vi "ReadParticleSizeSpectrum.vi"(1 "file path":path, 2 "Factor Size paramter":dbl=1.0) -> (0 "Particle Distribution Data":T1)   [LabVIEW 2013]
uses:
  ParticleDistributionData.ctl
  <vilib>/Platform/storage/lvStorage.llb/_openStorageWithRootAutoDetect.vi
  <vilib>/Platform/storage/lvStorage.llb/xStorage/xStorageSupp/ErrorOut.vi
  <vilib>/Platform/storage/lvStorage.llb/_queryPropPoly.vi
  <vilib>/Platform/storage/lvStorage.llb/_queryPropString.vi
  <vilib>/Platform/storage/lvStorage.llb/_queryGenericObjects.vi
  <vilib>/Platform/storage/lvStorage.llb/_loadAllDouble.vi
  <vilib>/Platform/storage/Storage.llb/Get Object Info.vi
  <vilib>/Platform/storage/Storage.llb/__closeStorageFromObject.vi
  <vilib>/imath/engines/lvmath2/RunTimeEngine/ErrorHandling/NIMS_Finalize Error.vi
  <vilib>/imath/engines/lvmath2/RunTimeEngine/IndexRead/NIMS M(S,$).vi
  <instcachedir>/0/NIMS M(S,$)_F24F360562DE41D8BE234322A2E15C65.lvgen/NIMS M(S,$)_F24F360562DE41D8BE234322A2E15C65_000.vi
  <vilib>/imathl/engines/lvmath/Functions/Error Handling/Create Error.vi
  <vilib>/imath/engines/lvmath2/RunTimeEngine/IndexRead/NIMS M(R2,$).vi
  <instcachedir>/0/NIMS M(R2,$)_AD8DC2FC79024024B2717E13B4A0EB4B.lvgen/NIMS M(R2,$)_AD8DC2FC79024024B2717E13B4A0EB4B_000.vi
  <vilib>/imath/engines/lvmath2/RunTimeEngine/NodeEndStatement/NIMS_NodeEndStatement_Output.vi
  <instcachedir>/0/NIMS_NodeEndStatement_Output_53EC0D466D134D7ABD903AC30B43404B.lvgen/NIMS_NodeEndStatement_Output_53EC0D466D134D7ABD903AC30B43404B_002.vi
  <instcachedir>/0/NIMS_NodeEndStatement_Output_53EC0D466D134D7ABD903AC30B43404B.lvgen/NIMS_NodeEndStatement_Output_53EC0D466D134D7ABD903AC30B43404B_005.vi
  <vilib>/Platform/storage/lvStorage.llb/xStorage/Open Data Storage/Open Data Storage.xnode
  <vilib>/Platform/storage/lvStorage.llb/xStorage/Read Data/Read Data.xnode
  <vilib>/Platform/storage/lvStorage.llb/xStorage/Close Data Storage/Close Data Storage.xnode
panel:
  in  "Particle Distribution Data 2":T1
  out "Double Charge Correction Flag":bool
  out "Concentration":dbl[][](array[numeric])
  out "Sizes":dbl[](array[numeric])
  out "error out":errorcluster
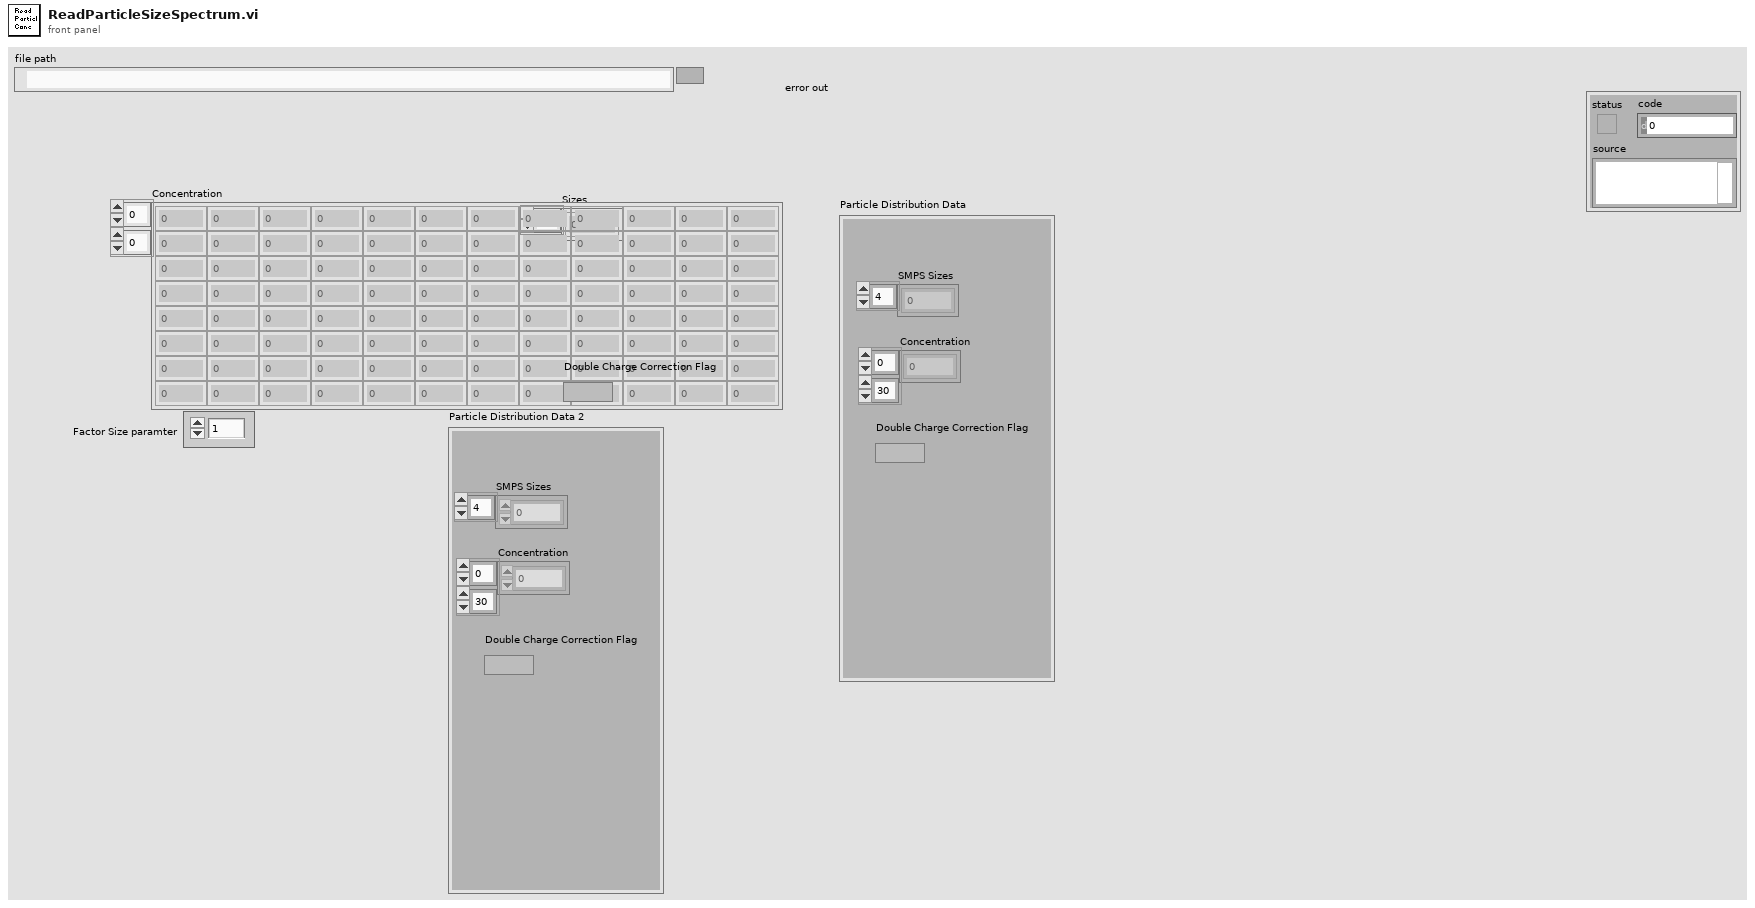
[diagram p1: front panel]
types:
  T1 = typedef "ParticleDistributionData.ctl" = cluster{"SMPS Sizes":dbl[], "Concentration":dbl[][], "Double Charge Correction Flag":bool}
  T2 = enum16{"open", "open or create", "create or replace", "create", "open (read only)"}
  T3 = enum16{"UPDATE", "READ", "QUERY", "CREATE CHILD", "CREATE", "CONNECT", "DISCONNECT"}
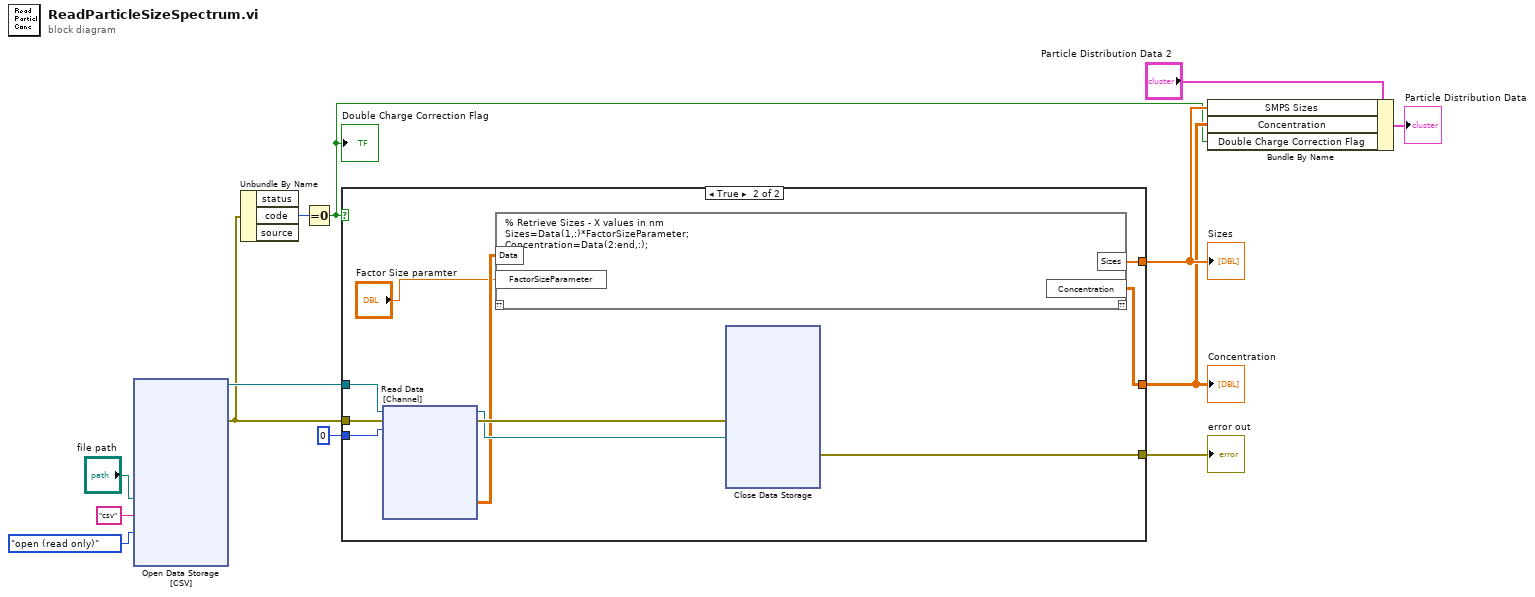
[diagram p0: block diagram]
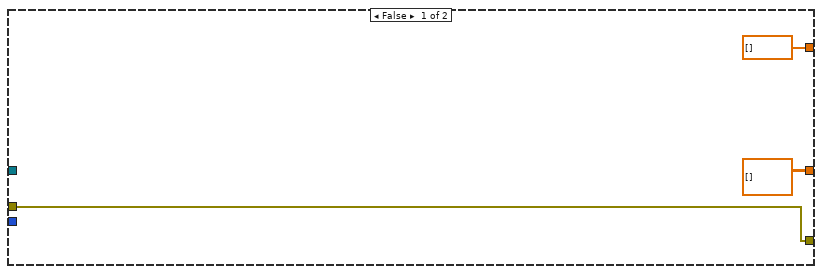
[diagram p2: hidden frame]
diagram:
  n1 = xnode "Open Data Storage\n[CSV]"("file path"="file path", "DataPlugin name"="csv", "function (open:0)"=T2."open (read only)") -> ("storage refnum (file)"=w13:refnum<k20>, "error out"=w7:errorcluster)  [unwired: 2 in, 1 out]
  n2 = Unbundle By Name(w7) -> ("code"=w6:i32)  [unwired: 2 out]
  n3 = Equal To 0?(x=w6) -> (x = 0?=w2:bool)
  "Double Charge Correction Flag" <- w2
  n4 = case shown="True" w2 {
    tunnel: w13 -> [_ w26]
    tunnel: [w16 w24] -> w12
    tunnel: 0 ("index") -> [_ w23]
    tunnel: [dbl[] [] ("Sizes") w20] -> w4
    tunnel: [dbl[][] [] ("Concentration") w19] -> w3
    tunnel: w7 -> [w16 w18]
    frame False {
    }
    frame True {
      n5 = xnode "Read Data\n[Channel]"("storage refnum (file)"=w26, "error in"=w18, "index"=w23) -> ("Signal"=w21:dbl[][], "storage refnum (file) out"=w22:refnum<k20>, "error out"=w25:errorcluster)  [unwired: 1 in, 1 out]
      n6 = mathscript code="% Retrieve Sizes - X values in nm\nSizes=Data(1,:)*FactorSizeParameter;\nConcentration=Data(2:end,:);"("Data"=w21, "FactorSizeParameter"="Factor Size paramter") -> ("Sizes"=w20:dbl[], "Concentration"=w19:dbl[][])  [unwired: 1 in, 1 out]
      n7 = xnode "Close Data Storage\n"("error in (no error)"=w25, "storage refnum (file)"=w22) -> ("error out"=w24:errorcluster)  [unwired: 1 out]
    }
  }
  "error out" <- w12
  "Sizes" <- w4
  "Concentration" <- w3
  n8 = Bundle By Name(cluster="Particle Distribution Data 2", "SMPS Sizes"=w4, "Concentration"=w3, "Double Charge Correction Flag"=w2) -> (→"Particle Distribution Data":T1)
